vi "Untitled 2.vi"() -> ()   [LabVIEW 2019]
uses:
  4f420df2-eb8c-479e-9334-d59b6ec1b998.vi
  <vilib>/JDP Science/JSONtext/Variant to JSON Text.vi
  <vilib>/JDP Science/JSONtext/LVClass Serializer/JSONtext LVClass Serializer.lvclass
  <vilib>/JDP Science/JSONtext/JSONtext.lvlib
panel:
  out "<JSON>":string
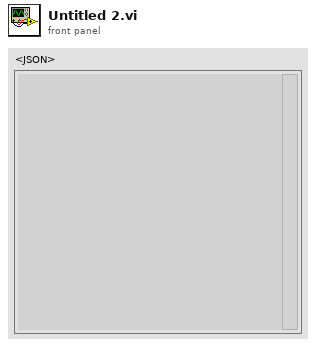
[diagram p1: front panel]
types:
  T1 = cluster{"AO Chassis Serial Number (i32)":string, "AO Channel (i32)":string, "AO Data (dbl)":string, "AO Sweeping? (bool)":string, "AI Chassis Serial Number (i32)":string, "AI Channel (i32)":string, "AI Data (dbl)":string, "AI Sweeping? (bool)":string, "MCLI Chassis Serial Number (i32)":string, "MCLI AI Channel (i32)":string, "MCLI Ref Channel (i32)":string, "MCLI X Data (dbl)":string, "MCLI Y Data (dbl)":string, "MCLC Sweeping? (bool)":string}
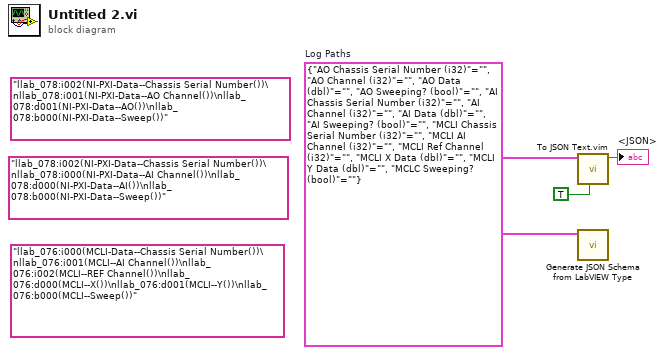
[diagram p0: block diagram]
diagram:
  w1 = T1 {"AO Chassis Serial Number (i32)"="", "AO Channel (i32)"="", "AO Data (dbl)"="", "AO Sweeping? (bool)"="", "AI Chassis Serial Number (i32)"="", "AI Channel (i32)"="", "AI Data (dbl)"="", "AI Sweeping? (bool)"="", "MCLI Chassis Serial Number (i32)"="", "MCLI AI Channel (i32)"="", "MCLI Ref Channel (i32)"="", "MCLI X Data (dbl)"="", "MCLI Y Data (dbl)"="", "MCLC Sweeping? (bool)"=""}  # Log Paths
  (unwired) "llab_078:i002(NI-PXI-Data--Chassis Serial Number())\nllab_078:i001(NI-PXI-Data--AO Channel())\nllab_078:d001(NI-PXI-Data--AO())\nllab_078:b000(NI-PXI-Data--Sweep())"
  (unwired) "llab_078:i002(NI-PXI-Data--Chassis Serial Number())\nllab_078:i000(NI-PXI-Data--AI Channel())\nllab_078:d000(NI-PXI-Data--AI())\nllab_078:b000(NI-PXI-Data--Sweep())"
  (unwired) "llab_076:i000(MCLI-Data--Chassis Serial Number())\nllab_076:i001(MCLI--AI Channel())\nllab_076:i002(MCLI--REF Channel())\nllab_076:d000(MCLI--X())\nllab_076:d001(MCLI--Y())\nllab_076:b000(MCLI--Sweep())"
  n1 = call "To JSON Text.vim"("Pretty Print?"=TRUE, "Anything"=w1) -> ("<JSON>"=→"<JSON>":string)  [unwired: 8 in, 1 out]
  n2 = call <vilib>:"Generate JSON Schema from LabVIEW Type.vi"("Variant"=w1) -> ()  [unwired: 9 in, 2 out]
